vi "getdbdataresults.vi"(5 "wheelname":string, 6 "connection reference":T2, 7 "runletter":string, 8 "ss ratio":u16(ring) items=["other", "36Cl"], 9 "holder":string, 10 "number of holders to calculate":dbl, 11 "charge state":i32=2) -> (0 "sample data list":T1, 1 "data":dbl[][](array[numeric]), 2 "sample data":string[][](array[string]), 3 "Array 2":dbl[][][](array[numeric]), 4 "connection reference out":T2)   [LabVIEW 2016]
uses:
  <vilib>/addons/database/Connection.llb/Conn ObjectReference.ctl
  <vilib>/Analysis/baseanly.llb/Mean (DBL).vi
  <vilib>/addons/database/Connection.llb/DB Tools Open Connec (String).vi
  <vilib>/addons/database/Connection.llb/Conn Execute.vi
  <vilib>/addons/database/Recordset.llb/Rec Fetch Recordset Data (R).vi
  <vilib>/addons/database/Recordset.llb/Rec Destroy - Connection.vi
  <vilib>/addons/database/NI_Database_API.lvlib
  <vilib>/Analysis/NI_AALBase.lvlib
panel:
  out "Array 9":dbl[][](array[numeric])
  out "element 2":i32
  out "appended array":dbl[](array[numeric])
  out "Array 6":dbl[](array[numeric])
  out "Array 8":dbl[](array[numeric])
  out "data 2":dbl[][](array[numeric])
  out "size(s)":i32[](array[numeric])
  out "output array":dbl[][](array[numeric])
  out "error out 4":errorcluster
  out "error out 3":errorcluster
  out "Array 7":dbl[](array[numeric])
  out "subarray 2":dbl[](array[numeric])
  out "Array 5":dbl[](array[numeric])
  out "Array 4":bool[](array[boolean])
  out "Array 3":bool[](array[boolean])
  out "element":dbl
  out "subarray":dbl[](array[numeric])
  out "Array":string[][](array[string])
  out "seq result":dbl
  in  "SQL query 2":string
  out "error out 2":errorcluster
  out "recordset data":variant[][](array[variant])
  out "error out":errorcluster
  in  "SQL query get data name":string="select distinct Position, holderid, samplename, userlast  from cycleresults where   runletter='2012al1' and wheelname='csv 5'  and sampletype<>'s' order by position;"
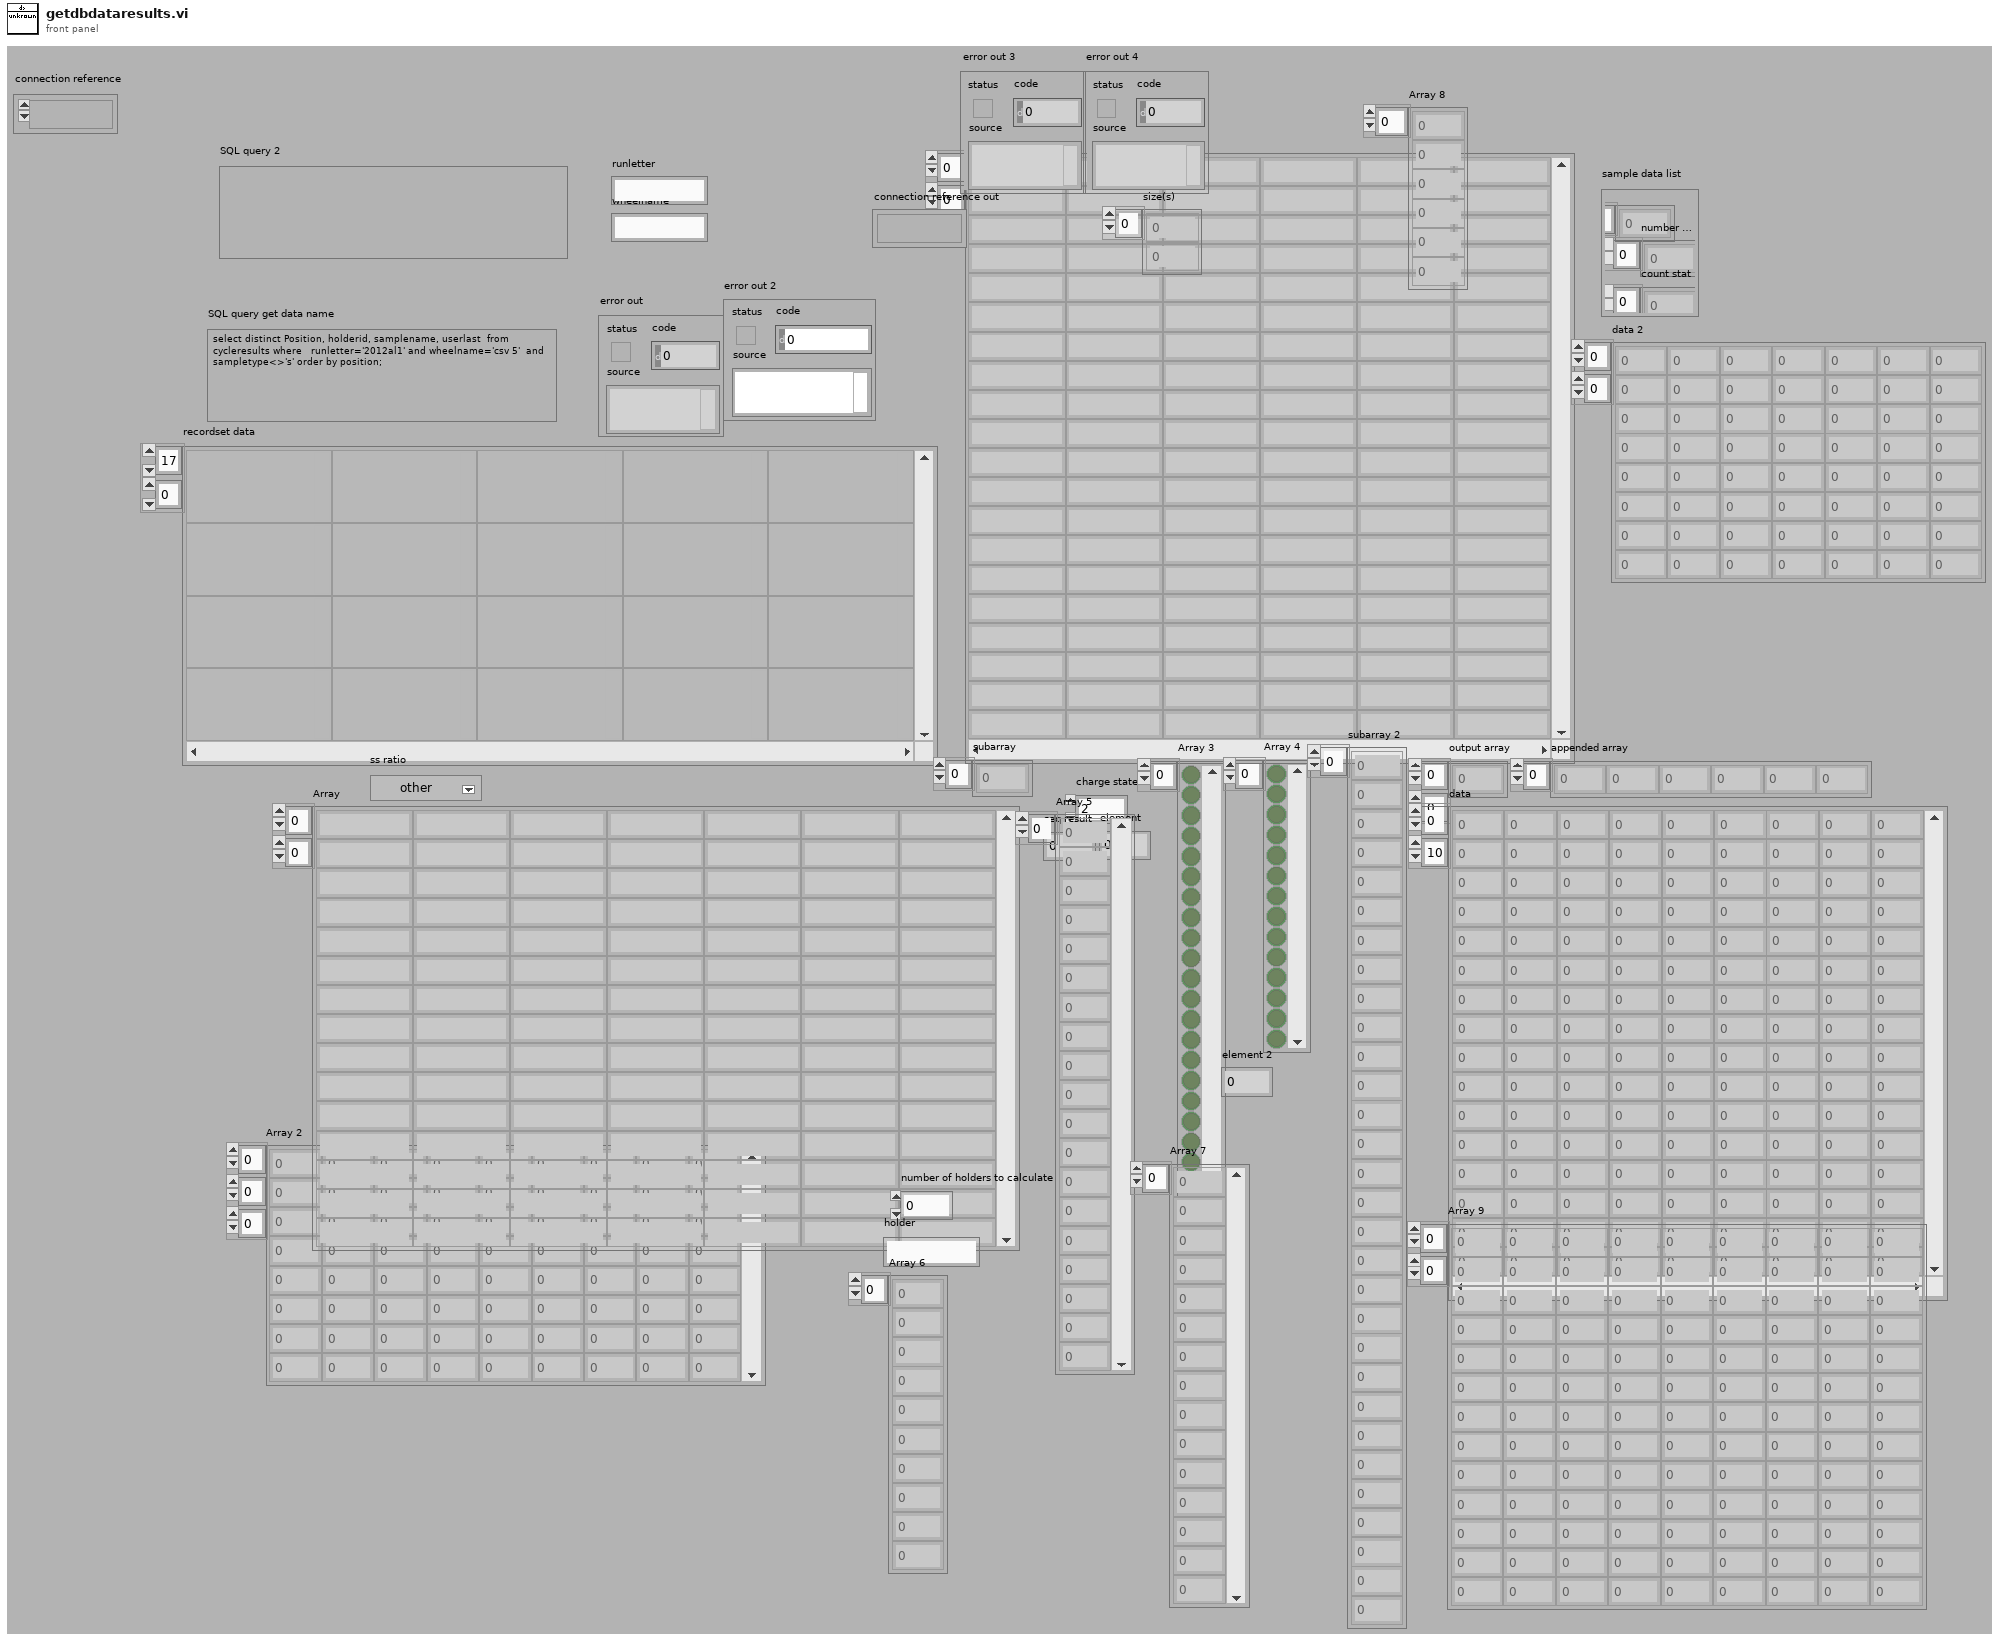
[diagram p1: front panel]
types:
  T1 = cluster{"last currents":dbl[], "number of cycles":i32[], "count stat":dbl[]}
  T2 = typedef "NI_Database_API.lvlib/Conn ObjectReference.ctl" = refnum<k1>
  T3 = typedef "NI_Database_API.lvlib/Rec ObjectReference.ctl" = refnum<k1>
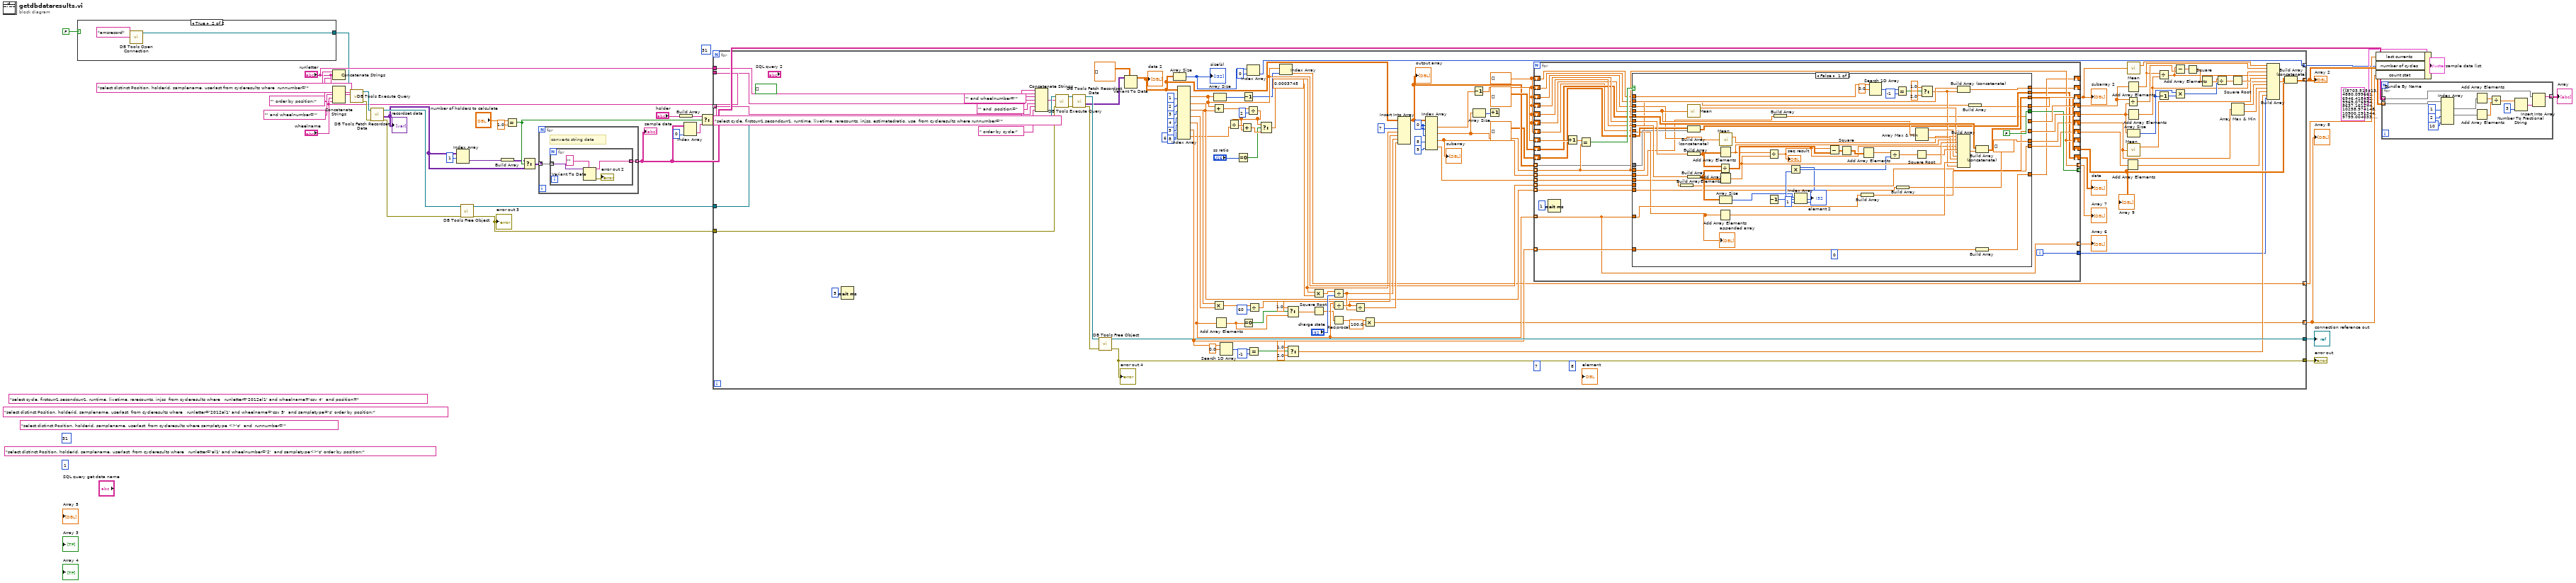
[diagram p0: block diagram]
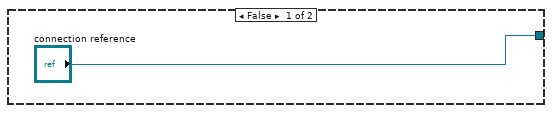
[diagram p2: hidden frame]
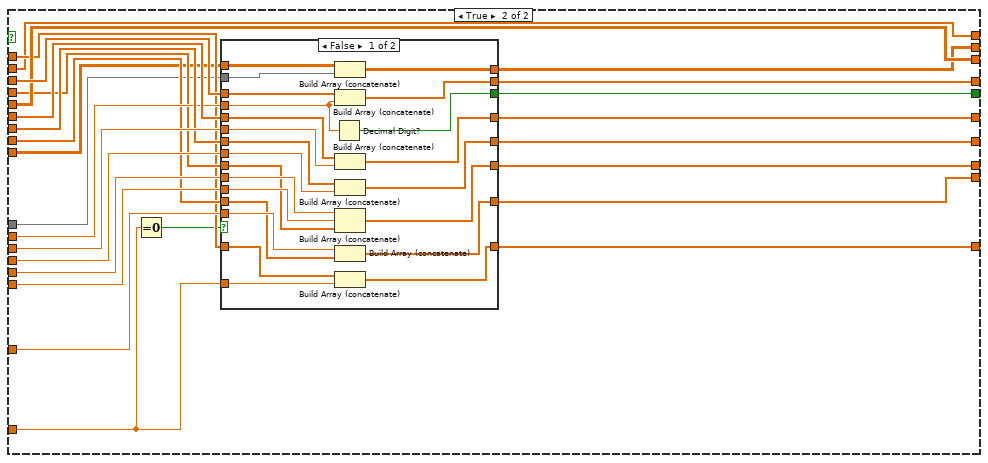
[diagram p3: hidden frame]
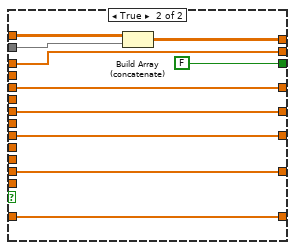
[diagram p4: hidden frame]
diagram:
  (unwired) "select distinct Position, holderid, samplename, userlast  from cycleresults where sampletype <>'s'  and  runnumber='" ("SQL query get data name")
  (unwired) 31
  (unwired) "select cycle, firstcurr1,secondcurr1, runtime, livetime, rarecounts, injss  from cycleresults where   runletter='2012al1' and wheelname='csv 4'  and position=" ("SQL query 3")
  w10 = "' order by position;" ("SQL query get data name")
  (unwired) "select distinct Position, holderid, samplename, userlast  from cycleresults where   runletter='2012al1' and wheelname='csv 5'  and sampletype='s' order by position;" ("SQL query get data name")
  w12 = "select distinct Position, holderid, samplename, userlast from cycleresults where  runnumber='" ("SQL query get data name")
  (unwired) "select distinct Position, holderid, samplename, userlast  from cycleresults where   runletter='al1' and wheelnumber='2'  and sampletype<>'s' order by position;" ("SQL query get data name")
  (unwired) 31
  (unwired) 1
  n1 = case shown="True" FALSE {
    tunnel: ["connection reference" w39] -> w1
    frame False {
    }
    frame True {
      n2 = call-poly <vilib>:"DB Tools Open Connection.vi"("connection information"="amsrecord") -> ("connection reference"=w39:T2)  [unwired: 7 in, 1 out]
    }
  }
  n3 = Concatenate Strings(w12, "runletter", w10) -> ()  [unwired: 1 out]
  n4 = Concatenate Strings(w12, "runletter", "' and wheelnumber='" ("SQL query get data name"), "wheelname", w10) -> (w9:string)
  n5 = call-poly <vilib>:"DB Tools Execute Query.vi"("SQL query"=w9, "connection reference"=w1) -> ("error out"=w37:errorcluster, "recordset reference"=w36:T3)  [unwired: 6 in]
  n6 = call-poly <vilib>:"DB Tools Fetch Recordset Data.vi"("error in (no error)"=w37, "recordset reference"=w36) -> ("error out"=w35:errorcluster, "recordset data"=w21:variant[][], "recordset reference out"=w34:T3)  [unwired: 3 in]
  "recordset data" <- w21
  n7 = Index Array(array=w21, index (row)=1) -> (element=w18:variant[])  [unwired: 1 in]
  n8 = call-poly <vilib>:"DB Tools Free Object.vi"("error in (no error)"=w35, "recordset reference"=w34) -> ("error out"=w31:errorcluster, "connection reference"=w32:T2)  [unwired: 8 in]
  "error out 3" <- w31
  n9 = Build Array(w18) -> (w17:variant[][])
  n10 = Equal?(x="number of holders to calculate", y=1.0) -> (x = y?=w22:bool)
  n11 = Select(t=w17, s=w22, f=w21) -> (s? t:f=w19:variant[][])
  n12 = for {
    tunnel: w19 -> [w42] mode=indexing
    tunnel: [w41] -> w30 mode=indexing
    # "converts string data"
    n13 = for {
      tunnel: w42 -> [w46] mode=indexing
      tunnel: [w44] -> w41 mode=indexing
      n14 = Variant To Data(type="", Variant=w46) -> (data=w44:string, error out=→"error out 2":errorcluster)  [unwired: 1 in]
    }
  }
  "sample data" <- w30
  n15 = Build Array("holder") -> (w23:string[])
  n16 = Index Array(array=w30, index (col)=0 ("disabled index (col)")) -> (element=w25:string[])  [unwired: 1 in]
  n17 = Select(t=w23, s=w22, f=w25) -> (s? t:f=w3:string[])
  n18 = for {
    tunnel: w3 -> [w101] mode=indexing
    tunnel: w31 -> [w159]
    tunnel: w32 -> [w158]
    tunnel: [w155] -> w15
    tunnel: [w154] -> w16
    tunnel: [w115] -> w28 mode=indexing
    tunnel: "runletter" -> [w103]
    tunnel: "wheelname" -> [w105]
    tunnel: [w79] -> w5 mode=indexing
    tunnel: [w77] -> w7 mode=indexing
    tunnel: [w67] -> w6 mode=indexing
    (unwired) 7
    (unwired) bool[] []
    w96 = dbl[] []
    w131 = 0 ("disabled index (col)")
    (unwired) 8 ("disabled index (col)")
    n19 = Wait (ms)(milliseconds to wait=u32 5) -> ()  [unwired: 1 out]
    n20 = Concatenate Strings("select cycle, firstcurr1,secondcurr1, runtime, livetime, rarecounts, injss, estimatedratio, use  from cycleresults where runnumber='" ("SQL query 3"), w103, "' and wheelnumber='" ("SQL query 3"), w105, "' and  position=" ("SQL query 3"), w101, " order by cycle;" ("string")) -> (w99:string)
    n21 = call-poly <vilib>:"DB Tools Execute Query.vi"("error in (no error)"=w159, "SQL query"=w99, "connection reference"=w158) -> ("error out"=w157:errorcluster, "recordset reference"=w161:T3)  [unwired: 5 in]
    n22 = call-poly <vilib>:"DB Tools Fetch Recordset Data.vi"("error in (no error)"=w157, "recordset reference"=w161) -> ("error out"=w156:errorcluster, "recordset data"=w153:variant[][], "recordset reference out"=w160:T3)  [unwired: 3 in]
    n23 = call-poly <vilib>:"DB Tools Free Object.vi"("error in (no error)"=w156, "recordset reference"=w160) -> ("error out"=w155:errorcluster, "connection reference"=w154:T2)  [unwired: 8 in]
    "error out 4" <- w155
    n24 = Variant To Data(type=dbl[][] [], Variant=w153) -> (data=w98:dbl[][])  [unwired: 1 in, 1 out]
    "data 2" <- w98
    n25 = Array Size(array=w98) -> (size(s)=w81:i32[])
    "size(s)" <- w81
    n26 = Index Array(array=w98, index (col) #1=1 ("index (row)"), index (col) #2=2 ("disabled index (col)"), index (col) #3=3 ("index (col)"), index (col) #4=4 ("index (col)"), index (col) #5=5 ("index (col)"), index (col) #6=8 ("index (col)"), index (col) #7=6 ("index (col)")) -> (element #1=w78:dbl[], element #2=w107:dbl[], element #3=w143:dbl[], element #4=w144:dbl[], element #5=w75:dbl[], element #6=w83:dbl[], element #7=w54:dbl[])  [unwired: 7 in]
    n27 = Add(x=w78, y=w107) -> (x+y=w53:dbl[])
    n28 = Multiply(x=w143, y=w144) -> (x*y=w136:dbl[])
    n29 = Array Size(array=w78) -> (size(s)=w66:i32)
    n30 = Add Array Elements(numeric array=w75) -> (sum=w72:dbl)
    n31 = Search 1D Array(1D array=w83, element=0.0) -> (index of element=w92:i32)  [unwired: 1 in]
    n32 = Equal To 0?(x="ss ratio") -> (x = 0?=w48:bool)
    n33 = Decrement(x=w66) -> (x-1=w76:i32)
    n34 = Equal To 0?(x=w72) -> (x = 0?=w74:bool)
    n35 = Divide(x=w53, y=2) -> (x/y=w51:dbl[])
    n36 = Divide(x=w51, y=w54) -> (x/y=w52:dbl[])
    n37 = Add(x=w52, y=w51) -> (x+y=w50:dbl[])
    n38 = Index Array(array=w81, index=0) -> (element=w79:i32)
    n39 = Equal?(x=w92, y=-1) -> (x = y?=w91:bool)
    n40 = Divide(x=w136, y=60) -> (x/y=w134:dbl[])
    n41 = Select(t=w51, s=w48, f=w50) -> (s? t:f=w47:dbl[])
    n42 = Index Array(array=w78, index=w76) -> (element=w77:dbl)
    n43 = Select(t=1.0, s=w74, f=w72) -> (s? t:f=w71:dbl)
    n44 = Select(t=1.0, s=w91, f=2.0) -> (s? t:f=w84:dbl)
    n45 = Multiply(x=w47, y=0.0003745) -> (x*y=w140:dbl[])
    n46 = Square Root(x=w71) -> (sqrt(x)=w70:dbl)
    n47 = Divide(x=w140, y="charge state") -> (x/y=w138:dbl[])
    n48 = Divide(x=w75, y=w134) -> (x/y=w139:dbl[])
    n49 = Reciprocal(x=w70) -> (1/x=w69:dbl)
    n50 = Divide(x=w139, y=w138) -> (x/y=w137:dbl[])
    n51 = Multiply(x=w69, y=100.0) -> (x*y=w67:dbl)
    n52 = Insert Into Array(array=w98, index (col)=7 ("disabled index (col)"), new element #1=w47, new element #2=w139, new element #3=w138, new element #4=w137) -> (w59:dbl[][])  [unwired: 1 in]
    "output array" <- w59
    n53 = Index Array(array=w59, index (row) #1=w131, index (col) #1=w131, index (col) #2=w131, index (col) #3=8 ("index (col)"), index (col) #4=9 ("index (col)")) -> (element #1=w130:dbl, element #2=w62:dbl[], element #3=w114:dbl[], element #4=w113:dbl[])  [unwired: 3 in]
    "subarray" <- w114
    n54 = Decrement(x=w130) -> (x-1=w129:dbl)
    n55 = Array Size(array=w62) -> (size(s)=w61:i32)
    n56 = Increment(x=w61) -> ()  [unwired: 1 out]
    n57 = for {
      tunnel: w62 -> [w179] mode=indexing
      tunnel: w114 -> [w191] mode=indexing
      tunnel: w113 -> [w190] mode=indexing
      shift-right: [w179] -> _
      shift-left: w129 -> [w193]
      shift-right: [w189] -> w65
      shift-left: w96 -> [w188]
      shift-right: [w186] -> w111
      shift-left: w96 -> [w185]
      shift-right: [w187] -> w112
      shift-left: w96 -> [w184]
      shift-right: [w183] -> w108
      shift-left: dbl[][] [] -> [w182]
      tunnel: [w181] -> _ mode=indexing
      tunnel: [w179] -> w110 mode=indexing
      tunnel: w78 -> [w178] mode=indexing
      tunnel: w107 -> [w177] mode=indexing
      shift-right: [w176] -> w89
      shift-left: w96 -> [w175]
      tunnel: w75 -> [w166] mode=indexing
      shift-right: [w174] -> w86
      shift-left: w96 -> [w173]
      tunnel: w83 -> [w172] mode=indexing
      shift-right: [w171] -> _
      shift-left: w96 -> [w170]
      shift-right: [w169] -> _
      shift-left: w96 -> [w168]
      tunnel: [w167] -> w82
      tunnel: [w166] -> w60 mode=indexing
      tunnel: w59 -> [w165] mode=indexing
      shift-right: [w164] -> w57
      shift-left: dbl[][] [] ("data") -> [w163]
      i -> [w167]
      n58 = Wait (ms)(milliseconds to wait=u32 1) -> ()  [unwired: 1 out]
      n59 = Increment(x=w193) -> (x+1=w180:dbl)
      n60 = Equal?(x=w180, y=w179) -> (x = y?=w192:bool)
      n61 = case shown="False" w192 {
        tunnel: w179 -> [w208 w265]
        tunnel: w191 -> [w200 w270]
        tunnel: w190 -> [w198 w271]
        tunnel: [w207 w274] -> w189
        tunnel: w188 -> [w204 w273]
        tunnel: [w197 w272] -> w187
        tunnel: [w199 w269] -> w186
        tunnel: w185 -> [w236 w268]
        tunnel: w184 -> [w235 w267]
        tunnel: [w247 w266] -> w183
        tunnel: w182 -> [w246 w266]
        tunnel: [FALSE w264] -> w181
        tunnel: w178 -> [_ w262]
        tunnel: w177 -> [w202 w263]
        tunnel: [w201 w261] -> w176
        tunnel: w175 -> [w231 w260]
        tunnel: w166 -> [w206 w259]
        tunnel: [w205 w258] -> w174
        tunnel: w173 -> [w203 w257]
        tunnel: w172 -> [w225 w253]
        tunnel: [w224 w256] -> w171
        tunnel: w170 -> [w223 w255]
        tunnel: [w219 w254] -> w169
        tunnel: w168 -> [w218 w254]
        tunnel: w165 -> [w210 w251]
        tunnel: [w209 w250] -> w164
        tunnel: w163 -> [w211 w249]
        frame False {
          (unwired) 0 ("index")
          (unwired) dbl[] []
          n62 = Build Array(w198) -> (w197:dbl[])
          n63 = call-poly <vilib>:"Mean.vi"("X"=w231) -> ("mean"=w232:dbl)  [unwired: 1 out]
          n64 = Build Array (concatenate)(w211, w210) -> (w209:dbl[][])
          n65 = Build Array(w236) -> (w234:dbl[][])
          n66 = Build Array(w235) -> (w233:dbl[][])
          n67 = Divide(x=w234, y=w233) -> (x/y=w245:dbl[][])
          n68 = Add Array Elements(numeric array=w203) -> (sum=w227:dbl)
          n69 = Add Array Elements(numeric array=w234) -> (sum=w228:dbl)
          n70 = Add Array Elements(numeric array=w233) -> (sum=w248:dbl)
          n71 = call-poly <vilib>:"Mean.vi"("X"=w204) -> ("mean"=w213:dbl)  [unwired: 1 out]
          n72 = Array Size(array=w233) -> (size(s)=w196:i32[])
          n73 = Divide(x=w228, y=w248) -> (x/y=w212:dbl)
          "seq result" <- w212
          n74 = Build Array(w200) -> (w199:dbl[])
          n75 = Index Array(array=w196, index=1) -> (element=w194:i32)
          "element 2" <- w194
          n76 = Decrement(x=w194) -> (x-1=w226:i32)
          n77 = Multiply(x=w194, y=w226) -> (x*y=w242:i32)
          n78 = Subtract(x=w212, y=w245) -> (x-y=w244:dbl[][])
          n79 = Square(x=w244) -> (x^2=w243:dbl[][])
          n80 = Build Array(w206) -> (w205:dbl[])
          n81 = Add Array Elements(numeric array=w243) -> (sum=w241:dbl)
          n82 = Search 1D Array(1D array=w223, element=0.0) -> (index of element=w221:i32)  [unwired: 1 in]
          n83 = Divide(x=w241, y=w242) -> (x/y=w240:dbl)
          n84 = Equal?(x=w221, y=-1) -> (x = y?=w217:bool)
          n85 = Build Array(w202) -> (w201:dbl[])
          n86 = Square Root(x=w240) -> (sqrt(x)=w239:dbl)
          n87 = Array Max & Min(array=w231) -> (max value=w230:dbl, min value=w229:dbl)  [unwired: 2 out]
          n88 = Select(t=1.0, s=w217, f=2.0) -> (s? t:f=w214:dbl)
          n89 = Build Array (concatenate)(w218, w214) -> (w219:dbl[])
          n90 = Build Array(w213, w228, w248, w212, w239, w232, w230, w229, w227, w214) -> (w238:dbl[])
          n91 = Build Array(w208) -> (w207:dbl[])
          n92 = Build Array (concatenate)(w246, w238) -> (w247:dbl[][])
          n93 = Build Array(w225) -> (w224:dbl[])
          "appended array" <- w203
        }
        frame True {
          n94 = Equal To 0?(x=w253) -> (x = 0?=w252:bool)
          n95 = case shown="False" w252 {
            tunnel: [w297 w304] -> w274
            tunnel: w273 -> [w279 w304]
            tunnel: [w296 w302] -> w272
            tunnel: w271 -> [w295 _]
            tunnel: w270 -> [w294 _]
            tunnel: [w293 w303] -> w269
            tunnel: w268 -> [w292 w303]
            tunnel: w267 -> [w291 w302]
            tunnel: w265 -> [w278 _]
            tunnel: [w290 FALSE] -> w264
            tunnel: w263 -> [w289 _]
            tunnel: w262 -> [w288 _]
            tunnel: [w287 w305] -> w261
            tunnel: w260 -> [w286 w305]
            tunnel: w259 -> [w285 _]
            tunnel: [w284 w306] -> w258
            tunnel: w257 -> [w283 w306]
            tunnel: [w282 w307] -> w256
            tunnel: w255 -> [w281 w307]
            tunnel: w253 -> [w280 _]
            tunnel: w251 -> [w277 w299]
            tunnel: [w276 w298] -> w250
            tunnel: w249 -> [w275 w300]
            frame False {
              n96 = Decimal Digit?(1:w278) -> (0:w290:bool)
              n97 = Build Array (concatenate)(w275, w277) -> (w276:dbl[][])
              n98 = Build Array (concatenate)(w279, w278) -> (w297:dbl[])
              n99 = Build Array (concatenate)(w292, w294) -> (w293:dbl[])
              n100 = Build Array (concatenate)(w291, w295) -> (w296:dbl[])
              n101 = Build Array (concatenate)(w288, w289, w286) -> (w287:dbl[])
              n102 = Build Array (concatenate)(w285, w283) -> (w284:dbl[])
              n103 = Build Array (concatenate)(w281, w280) -> (w282:dbl[])
            }
            frame True {
              n104 = Build Array (concatenate)(w300, w299) -> (w298:dbl[][])
            }
          }
        }
      }
    }
    "subarray 2" <- w65
    "Array 7" <- w110
    "Array 6" <- w60
    "data" <- w57
    "Array 9" <- w108
    n105 = Divide(x=w111, y=w112) -> (x/y=w119:dbl[])
    n106 = Add Array Elements(numeric array=w86) -> (sum=w85:dbl)
    n107 = Add Array Elements(numeric array=w111) -> (sum=w117:dbl)
    n108 = Add Array Elements(numeric array=w112) -> (sum=w118:dbl)
    n109 = call-poly <vilib>:"Mean.vi"("X"=w65) -> ("mean"=w64:dbl)  [unwired: 1 out]
    n110 = Array Size(array=w112) -> (size(s)=w123:i32)
    n111 = call-poly <vilib>:"Mean.vi"("X"=w89) -> ("mean"=w63:dbl)  [unwired: 1 out]
    n112 = Divide(x=w117, y=w118) -> (x/y=w116:dbl)
    n113 = Decrement(x=w123) -> (x-1=w122:i32)
    n114 = Subtract(x=w116, y=w119) -> (x-y=w120:dbl[])
    n115 = Multiply(x=w123, y=w122) -> (x*y=w124:i32)
    n116 = Square(x=w120) -> (x^2=w121:dbl[])
    n117 = Add Array Elements(numeric array=w121) -> (sum=w125:dbl)
    n118 = Divide(x=w125, y=w124) -> (x/y=w126:dbl)
    n119 = Square Root(x=w126) -> (sqrt(x)=w127:dbl)
    n120 = Array Max & Min(array=w89) -> (max value=w88:dbl, min value=w87:dbl)  [unwired: 2 out]
    n121 = Build Array(w64, w117, w118, w116, w127, w63, w88, w87, w85, w84, w82) -> (w109:dbl[])
    n122 = Build Array (concatenate)(w108, w109) -> (w115:dbl[][])
  }
  "error out" <- w15
  "Array 2" <- w28
  "connection reference out" <- w16
  "Array 8" <- w6
  n123 = Bundle By Name(cluster=T1 {"last currents"=[8703.515413, 4880.099661, 6946.418452, 9969.076994, 8637.161244, 10258.974148, 10900.291344, 9799.004033, 10334.991583, 10428.403026], "number of cycles"=[4, 4, 4, 4, 4, 4, 4, 8, 8, 13], "count stat"=[]} ("sample data list"), "last currents"=w7, "number of cycles"=w5, "count stat"=w6) -> (→"sample data list":T1)
  n124 = for {
    tunnel: w28 -> [w320] mode=indexing
    tunnel: w30 -> [w311] mode=indexing
    tunnel: [w308] -> w29 mode=indexing
    n125 = Index Array(array=w320, index (col) #1=1 ("disabled index (col)"), index (col) #2=2 ("index (col)"), index (col) #3=10 ("index (col)")) -> (element #1=w316:dbl[], element #2=w317:dbl[])  [unwired: 3 in, 1 out]
    n126 = Add Array Elements(numeric array=w316) -> (sum=w314:dbl)
    n127 = Add Array Elements(numeric array=w317) -> (sum=w315:dbl)
    n128 = Divide(x=w314, y=w315) -> (x/y=w313:dbl)
    n129 = Number To Fractional String(number=w313, precision (6)=i16 3) -> (F-format string=w310:string)  [unwired: 2 in]
    n130 = Insert Into Array(array=w311, new element=w310) -> (w308:string[])  [unwired: 1 in]
  }
  "Array" <- w29
